vi "S2C_FORNAX_Proc_LoadViperScript.vi"(8 "Error In":errorcluster) -> (0 "Error Out":errorcluster)   [LabVIEW 2015]
doc: "Find the parameters associated with a Fornax command, given the command index."
uses:
  S2C_FORNAX_Proc_Globals.vi
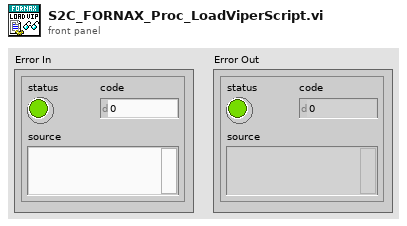
[diagram p1: front panel]
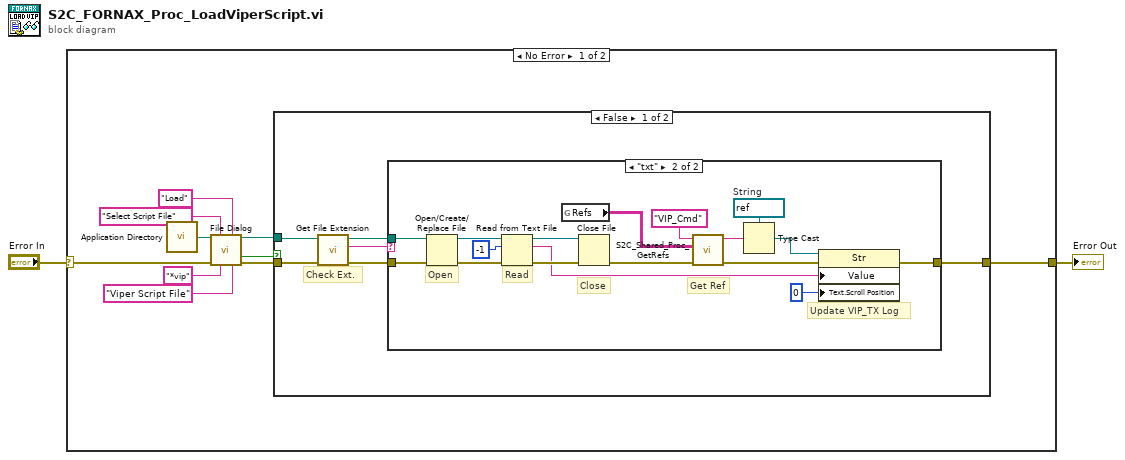
[diagram p0: block diagram]
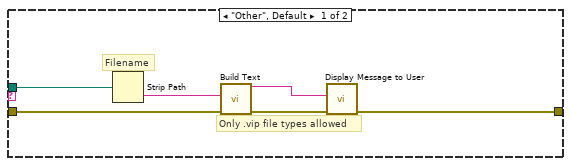
[diagram p2: hidden frame]
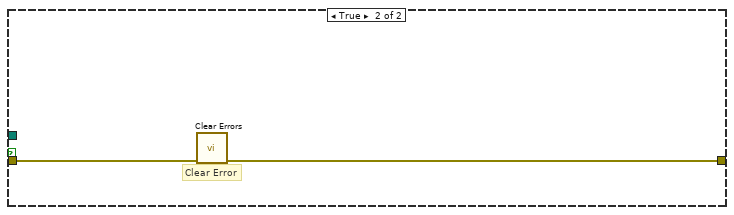
[diagram p3: hidden frame]
diagram:
  n1 = case shown="No Error" "Error In" {
    selector: "Error In" -> [w8 w44]
    tunnel: [w4 w44] -> w1
    frame No Error {
      n2 = call <vilib>:"Application Directory.vi"() -> ("Application Directory"=w7:path)
      n3 = call "File Dialog"("start path"=w7, "prompt"="Select Script File", "button label"="Load", "error in"=w8, "pattern (all files)"="*vip", "pattern label"="Viper Script File") -> ("selected path"=w3:path, "cancelled"=w5:bool, "error out"=w6:errorcluster)  [unwired: 6 in, 1 out]
      n4 = case shown="False" w5 {
        tunnel: w6 -> [w16 w43]
        tunnel: [w18 w42] -> w4
        tunnel: w3 -> [w15 _]
        frame False {
          # "Check Ext."
          n5 = call <vilib>:"Get File Extension.vi"("error in (no error)"=w16, "file"=w15) -> ("error out"=w13:errorcluster, "lowercase file extension"=w17:string, "dup file"=w14:path)  [unwired: 5 in, 2 out]
          n6 = case shown="\"txt\"" w17 {
            tunnel: w13 -> [w24 w41]
            tunnel: w14 -> [w21 w40]
            tunnel: [w22 w25] -> w18
            frame "Other", Default {
              # "Filename"
              # "Only .vip file types allowed"
              n7 = Strip Path(path=w21) -> (name=w20:string)  [unwired: 1 out]
              n8 = call "Build Text"("File"=w20, "error in (no error)"=w24) -> ("Result"=w19:string, "error out"=w23:errorcluster)  [unwired: 12 in]
              n9 = call "Display Message to User"("error in (no error)"=w23, "Message"=w19) -> ("error out"=w22:errorcluster)  [unwired: 8 in, 1 out]
            }
            frame "txt" {
              w31 = refnum<vi> refnum  # String
              # "Get Ref"
              # "Update VIP_TX Log"
              # "Close"
              # "Read"
              # "Open"
              n10 = Open/Create/Replace File(file path (use dialog)=w40, error in=w41) -> (refnum out=w38:refnum<file>, error out=w39:errorcluster)  [unwired: 4 in, 1 out]
              n11 = Read from Text File(file (use dialog)=w38, count=-1, error in=w39) -> (refnum out=w35:refnum<file>, text=w26:string, error out=w36:errorcluster)  [unwired: 1 in, 1 out]
              n12 = global read "S2C_FORNAX_Proc_Globals.vi" "Refs"() -> (w33:string[][])
              n13 = Close File(refnum=w35, error in=w36) -> (error out=w34:errorcluster)  [unwired: 1 out]
              n14 = call "S2C_Shared_Proc_GetRefs.vi"("Error In"=w34, "Refs"=w33, "Label"="VIP_Cmd") -> ("Error Out"=w28:errorcluster, "Reference"=w27:string)  [unwired: 7 in]
              n15 = Type Cast(type=w31, x=w27) -> (*(type *) &x=w29:refnum<vi>)
              n16 = property on="Property Node" class="Str"(reference=w29, error in=w28, "Value"=w26, "Text.Scroll Position"=u32 0) -> (error out=w25:errorcluster)  [unwired: 1 out]
            }
          }
        }
        frame True {
          # "Clear Error"
          n17 = call <vilib>:"Clear Errors.vi"("error in (no error)"=w43) -> ("error out"=w42:errorcluster)  [unwired: 5 in, 1 out]
        }
      }
    }
    frame Error {
    }
  }
  "Error Out" <- w1
